vi "Counter_init.vi"() -> (0 "ErrMsg":string)   [LabVIEW 2010]
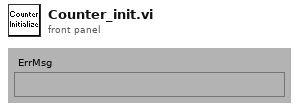
[diagram p1: front panel]
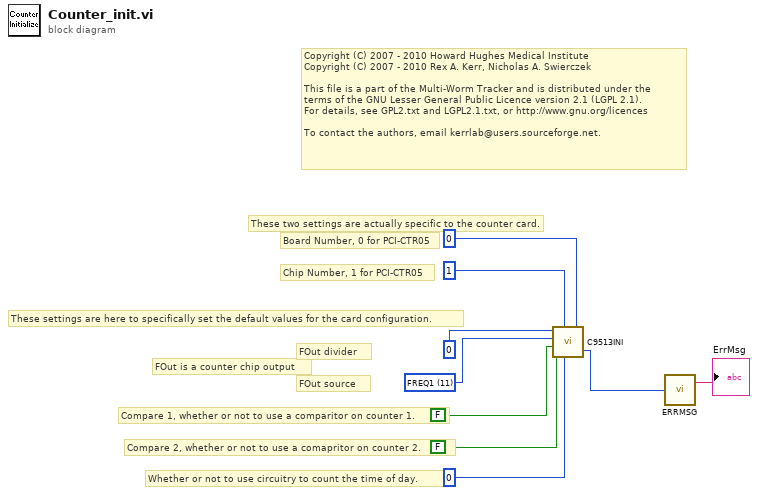
[diagram p0: block diagram]
diagram:
  w6 = u32 11 items=["TCPREVCTR", "CTRINPUT1", "CTRINPUT2", "CTRINPUT3", "CTRINPUT4", "CTRINPUT5", "GATE1", "GATE2", "GATE3", "GATE4", "GATE5", "FREQ1", "FREQ2", "FREQ3", "FREQ4", "FREQ5", "CTRINPUT6", "CTRINPUT7", "CTRINPUT8", "CTRINPUT9", "CTRINPUT10", "GATE6", "GATE7", "GATE8", "GATE9", "GATE10", "FREQ6", "FREQ7", "FREQ8", "FREQ9", "FREQ10", "CTRINPUT11", "CTRINPUT12", "CTRINPUT13", "CTRINPUT14", "CTRINPUT15", "GATE11", "GATE12", "GATE13", "GATE14", "GATE15", "FREQ11", "FREQ12", "FREQ13", "FREQ14", "FREQ15", "CTRINPUT16", "CTRINPUT17", "CTRINPUT18", "CTRINPUT19", "CTRINPUT20", "GATE16", "GATE17", "GATE18", "GATE19", "GATE20", "FREQ16", "FREQ17", "FREQ18", "FREQ19", "FREQ20"] ("FOut Source")
  # "Copyright (C) 2007 - 2010 Howard Hughes Medical Institute\nCopyright (C) 2007 - 2010 Rex A. Kerr, Nicholas A. Swierczek\n \nThis file is a part of the Multi-Worm Tracker and is distributed under the\nterms of the GNU Lesser General Public Licence version 2.1 (LGPL 2.1).\nFor details, see GPL2.txt and LGPL2.1.txt, or http://www.gnu.org/licences\n \nTo contact the authors, email kerrlab@users.sourceforge.net."
  # "FOut is a counter chip output"
  # "These settings are here to specifically set the default values for the card configuration."
  # "These two settings are actually specific to the counter card."
  # "Whether or not to use circuitry to count the time of day."
  # "Compare 2, whether or not to use a comapritor on counter 2."
  # "Compare 1, whether or not to use a comparitor on counter 1."
  # "FOut source"
  # "FOut divider"
  # "Chip Number, 1 for PCI-CTR05"
  # "Board Number, 0 for PCI-CTR05"
  n1 = call <menus>:"C9513INI.VI"("BoardNum (0)"=u32 0, "TimeOfDay (0)"=u32 0, "ChipNum (1)"=u32 1, "Compare2 (disabled)"=FALSE, "Compare1 (disabled)"=FALSE, "FOut Source"=w6, "FOutDivider"=u32 0) -> ("ErrCode"=w2:i32)
  n2 = call <menus>:"ERRMSG.VI"("ErrCode"=w2) -> ("ErrMsg"=→"ErrMsg":string)  [unwired: 1 out]
